vi "Generic Boundary DAO.vi"(5 "Section":string, 7 "refnum in":T1, 8 "error in (no error)":errorcluster, 10 "Limit Boundary Parameters In":T3, 11 "Persistent DAO Actions":T2) -> (0 "error out":errorcluster, 2 "Limit Boundary Parameters Out":T3, 4 "refnum out":T1)   [LabVIEW 2009]
uses:
  Limit Boundary Parameters.ctl
  Metadata/Persistant DAO Actions.ctl
  <vilib>/Utility/config.llb/Config Data RefNum.ctl
  <vilib>/Utility/config.llb/Read Key (String).vi
  <vilib>/Utility/config.llb/Read Key (Double).vi
  <vilib>/Utility/config.llb/Write Key (String).vi
  <vilib>/Utility/config.llb/Write Key (Double).vi
  <vilib>/Utility/config.llb/NI_LVConfig.lvlib
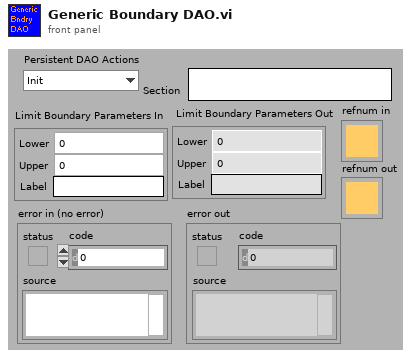
[diagram p1: front panel]
types:
  T1 = typedef "NI_LVConfig.lvlib/Config Data RefNum.ctl" = refnum<k1>
  T2 = typedef "Persistant DAO Actions.ctl" = enum16{"Init", "Get", "Set", "Load", "Save"}
  T3 = typedef "Limit Boundary Parameters.ctl" = cluster{"Lower":dbl, "Upper":dbl, "Label":string}
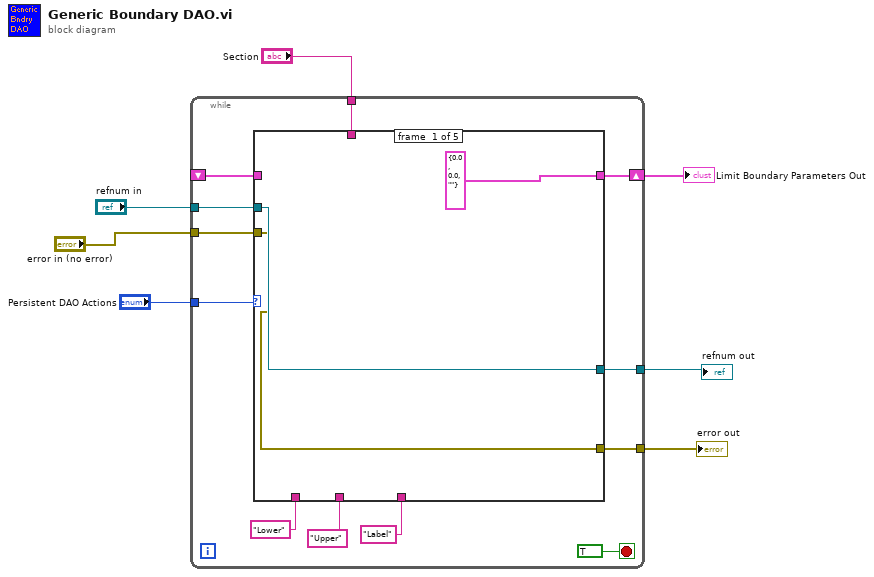
[diagram p0: block diagram]
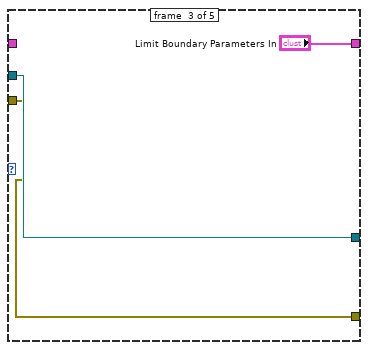
[diagram p3: hidden frame]
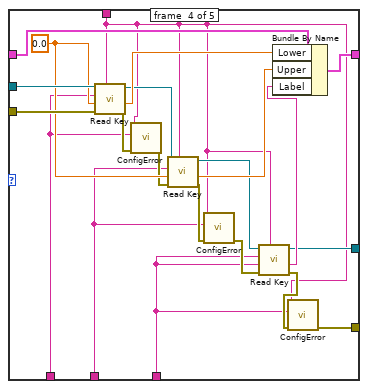
[diagram p4: hidden frame]
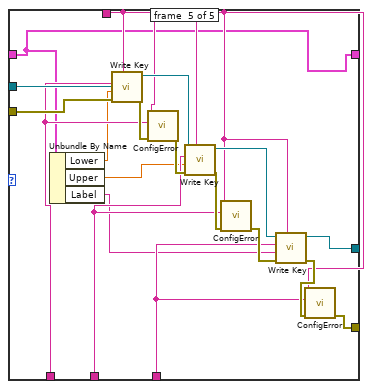
[diagram p5: hidden frame]
diagram:
  n1 = while {
    tunnel: "Persistent DAO Actions" -> [w18]
    shift-right: [w17] -> w6
    shift-left: _ -> [w16]
    tunnel: "Section" -> [w15]
    tunnel: "refnum in" -> [w14]
    tunnel: "error in (no error)" -> [w13]
    tunnel: [w9] -> w2
    tunnel: [w8] -> w1
    stop <- TRUE stop-if-true
    n2 = case shown="\"Load\"" w18 {
      tunnel: [T3 {"Lower"=0.0, "Upper"=0.0, "Label"=""} ("Limit Boundary Parameters In") w25 "Limit Boundary Parameters In" w47 w53] -> w17
      tunnel: w16 -> [_ w25 _ w46 w53]
      tunnel: w15 -> [_ _ _ w29 w54]
      tunnel: w14 -> [w21 w24 w27 w49 w68]
      tunnel: w13 -> [w20 w23 w26 w48 w67]
      tunnel: "Lower" ("key") -> [_ _ _ w40 w64]
      tunnel: "Upper" ("key") -> [_ _ _ w37 w61]
      tunnel: "Label" ("key") -> [_ _ _ w30 w55]
      tunnel: [w21 w24 w27 w33 w58] -> w9
      tunnel: [w20 w23 w26 w31 w56] -> w8
      frame #0 {
      }
      frame #1 {
      }
      frame #2 {
      }
      frame #3 {
        w43 = 0.0
        n3 = call-poly <vilib>:"Read Key.vi"("section"=w29, "error in (no error)"=w48, "default value"=w43, "key"=w40, "refnum"=w49) -> ("error out"=w41:errorcluster, "value"=w45:dbl, "refnum out"=w44:T1)  [unwired: 4 out]
        n4 = call "ConfigError.vi"("error in (no error)"=w41, "Key"=w40, "Section"=w29) -> ("error out"=w39:errorcluster)  [unwired: 8 out]
        n5 = call-poly <vilib>:"Read Key.vi"("section"=w29, "error in (no error)"=w39, "default value"=w43, "key"=w37, "refnum"=w44) -> ("error out"=w38:errorcluster, "value"=w42:dbl, "refnum out"=w35:T1)  [unwired: 4 out]
        n6 = call "ConfigError.vi"("error in (no error)"=w38, "Key"=w37, "Section"=w29) -> ("error out"=w36:errorcluster)  [unwired: 8 out]
        n7 = call-poly <vilib>:"Read Key.vi"("section"=w29, "error in (no error)"=w36, "default value"=w30, "key"=w30, "refnum"=w35) -> ("error out"=w32:errorcluster, "value"=w34:string, "refnum out"=w33:T1)  [unwired: 1 in, 3 out]
        n8 = Bundle By Name(cluster=w46, "Lower"=w45, "Upper"=w42, "Label"=w34) -> (w47:T3)
        n9 = call "ConfigError.vi"("error in (no error)"=w32, "Key"=w30, "Section"=w29) -> ("error out"=w31:errorcluster)  [unwired: 8 out]
      }
      frame #4 {
        n10 = Unbundle By Name(w53) -> ("Lower"=w52:dbl, "Upper"=w51:dbl, "Label"=w50:string)
        n11 = call-poly <vilib>:"Write Key.vi"("section"=w54, "error in (no error)"=w67, "value"=w52, "key"=w64, "refnum"=w68) -> ("error out"=w65:errorcluster, "refnum out"=w66:T1)  [unwired: 3 in, 2 out]
        n12 = call "ConfigError.vi"("error in (no error)"=w65, "Key"=w64, "Section"=w54) -> ("error out"=w63:errorcluster)  [unwired: 8 out]
        n13 = call-poly <vilib>:"Write Key.vi"("section"=w54, "error in (no error)"=w63, "value"=w51, "key"=w61, "refnum"=w66) -> ("error out"=w62:errorcluster, "refnum out"=w59:T1)  [unwired: 3 in, 2 out]
        n14 = call "ConfigError.vi"("error in (no error)"=w62, "Key"=w61, "Section"=w54) -> ("error out"=w60:errorcluster)  [unwired: 8 out]
        n15 = call-poly <vilib>:"Write Key.vi"("section"=w54, "error in (no error)"=w60, "value"=w50, "key"=w55, "refnum"=w59) -> ("error out"=w57:errorcluster, "refnum out"=w58:T1)  [unwired: 1 in, 4 out]
        n16 = call "ConfigError.vi"("error in (no error)"=w57, "Key"=w55, "Section"=w54) -> ("error out"=w56:errorcluster)  [unwired: 8 out]
      }
    }
  }
  "Limit Boundary Parameters Out" <- w6
  "error out" <- w1
  "refnum out" <- w2
